vi "Set Separate Compiled Code for VIs in a Folder.vi"(8 "error in (no error)":errorcluster, 10 "Separate Compiled Code? (T)":bool=TRUE, 11 "VI Folder":path) -> (0 "error out":errorcluster, 3 "VI List":path[](array[path]))   [LabVIEW 2016, in "SLL Scripting.lvlib"]
doc: "This is used to set/unset the \"Separate Compiled Code\" option for all VIs in the specified folder."
uses:
  SLL Scripting.lvlib
panel:
  out "Progress":i32
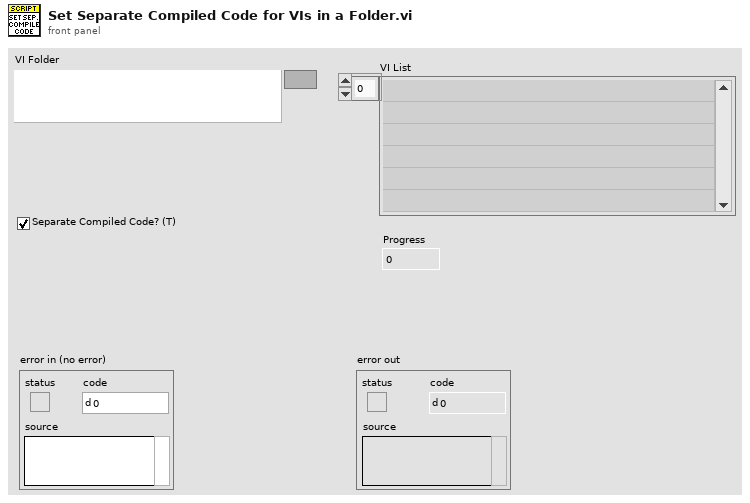
[diagram p1: front panel]
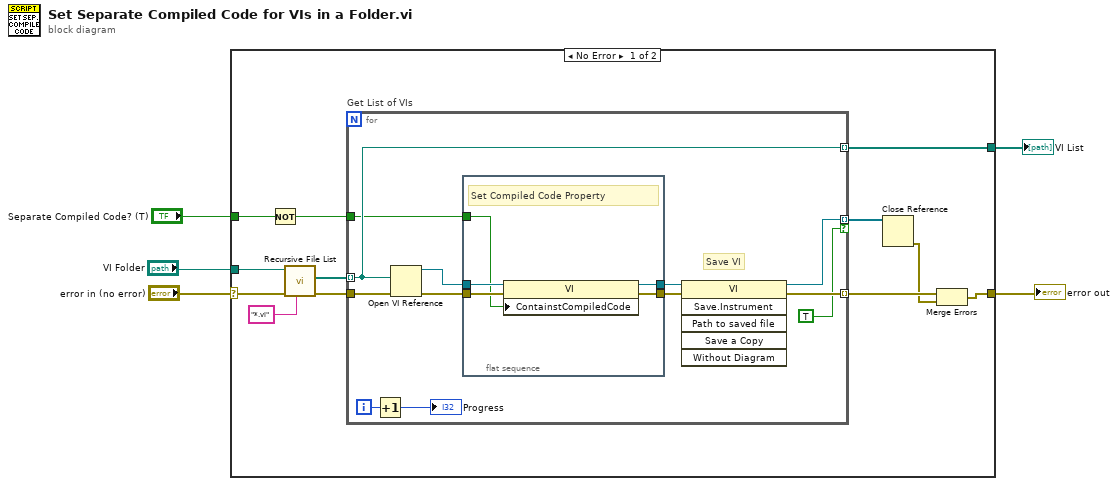
[diagram p0: block diagram]
diagram:
  n1 = case shown="No Error" "error in (no error)" {
    selector: "error in (no error)" -> [w12 w35]
    tunnel: "VI Folder" -> [w16 _]
    tunnel: [w13 _] -> w4
    tunnel: [w8 w35] -> w2
    tunnel: "Separate Compiled Code? (T)" -> [w7 _]
    frame No Error {
      n2 = Not(x=w7) -> (.not. x?=w6:bool)
      n3 = call <vilib>:"Recursive File List.vi"("pattern"="*.vi", "error in (no error)"=w12, "Folder Path"=w16) -> ("error out"=w11:errorcluster, "All Files in Dir"=w14:path[])  [unwired: 4 in, 3 out]
      n4 = for "Get List of VIs" {
        tunnel: [w27] -> w17 mode=indexing if=TRUE
        tunnel: w14 -> [w24] mode=indexing
        tunnel: [w24] -> w13 mode=indexing
        tunnel: w11 -> [w26]
        tunnel: [w28] -> w10 mode=indexing
        tunnel: w6 -> [w23]
        i -> [w29]
        # "Save VI"
        n5 = Increment(x=w29) -> (x+1=→"Progress":i32)
        n6 = Open VI Reference(vi path=w24, error in (no error)=w26) -> (vi reference=w22:refnum<vi>, error out=w21:errorcluster)  [unwired: 4 in]
        n7 = flat-sequence {
          tunnel: w22 -> [w32]
          tunnel: w21 -> [w34]
          tunnel: [w33] -> w20
          tunnel: [w31] -> w19
          tunnel: w23 -> [w30]
          frame #0 {
            # "Set Compiled Code Property"
            n8 = property class="VI"(reference=w32, error in=w34, "ContainstCompiledCode"=w30) -> (reference out=w31:refnum<vi>, error out=w33:errorcluster)
          }
        }
        n9 = invoke class="VI" method="Save.Instrument"(reference=w19, error in=w20) -> (reference out=w27:refnum<vi>, error out=w28:errorcluster)  [unwired: 4 in, 4 out]
      }
      n10 = Close Reference(reference=w17) -> (error out=w9:errorcluster)  [unwired: 1 in]
      n11 = Merge Errors(w10, w9) -> (w8:errorcluster)
    }
    frame Error {
    }
  }
  "error out" <- w2
  "VI List" <- w4
